vi "Measurement Template.vi"(8 "error in (no error)":errorcluster, 10 "stop":bool, 11 "measurement configuration":cluster{}) -> (0 "error out":errorcluster, 3 "measurement results":cluster{})   [LabVIEW 2021]
uses:
  <vilib>/gRPC/LabVIEW gRPC Library/grpc-lvsupport-release.lvlib
  Runtime/Clients/Measurement Service Client V2/Measurement Service Client V2.lvlib
  35f71eb9-7158-4110-bfb1-6d749e6fa8f4.vi
  Runtime/Clients/Measurement Client V2/Client.lvlib
  ef0035e8-05ef-469b-9be2-5e457b1f40d8.vi
  Runtime/Clients/Measurement Service Client V2/RPC Messages/ni_measurementlink_measurement_v2_MeasureRequest.ctl
  Runtime/Clients/Measurement Service Client V2/RPC Messages/ni_measurementlink_PinMapContext.ctl
  Runtime/Clients/Measurement Service Client V2/RPC Messages/google_protobuf_Any.ctl
panel:
  in  "service class":string="Voltage Measurement_LabVIEW"
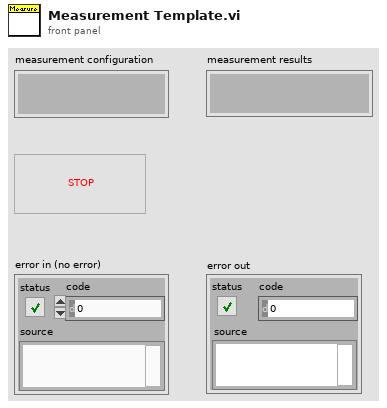
[diagram p1: front panel]
types:
  T1 = typedef "Measurement Service Client V2.lvlib/ni_measurementlink_measurement_v2_MeasureRequest.ctl" = cluster{"configuration_parameters":T2, "pin_map_context":T3}
  T2 = typedef "Measurement Service Client V2.lvlib/google_protobuf_Any.ctl" = cluster{"type_url":string, "value":u8[]}
  T3 = typedef "Measurement Service Client V2.lvlib/ni_measurementlink_PinMapContext.ctl" = cluster{"pin_map_id":string, "sites":i32[]}
  T4 = typedef "grpc-lvsupport-release.lvlib/grpcId.ctl" = u64
  T5 = typedef "grpc-lvsupport-release.lvlib/Message Metadata.ctl" = cluster{"Version":i32, "Name":string, "Type Url":string, "Elements":T6[], "Has Oneof":bool}
  T6 = typedef "grpc-lvsupport-release.lvlib/Message Element Metadata.ctl" = cluster{"Field Name":string, "Embedded Message Name":string, "Protobuf Index":i32, "MessageElementType":T7, "Repeated":bool, "Is in Oneof":bool, "Oneof Container Name":string}
  T7 = typedef "grpc-lvsupport-release.lvlib/Message Element Type.ctl" = enum32{"Int32Value", "FloatValue", "DoubleValue", "BoolValue", "StringValue", "MessageValue", "Int64Value", "UInt32Value", "UInt64Value", "EnumValue", "Bytes", "Fixed64", "Fixed32", "SFixed64", "SFixed32", "SInt64", "SInt32"}
  T8 = typedef "grpc-lvsupport-release.lvlib/Any.ctl" = cluster{"Type Url":string, "Bytes":u8[]}
  T9 = typedef "Measurement Service Client V2.lvlib/ni_measurementlink_measurement_v2_MeasureResponse.ctl" = cluster{"outputs":T2}
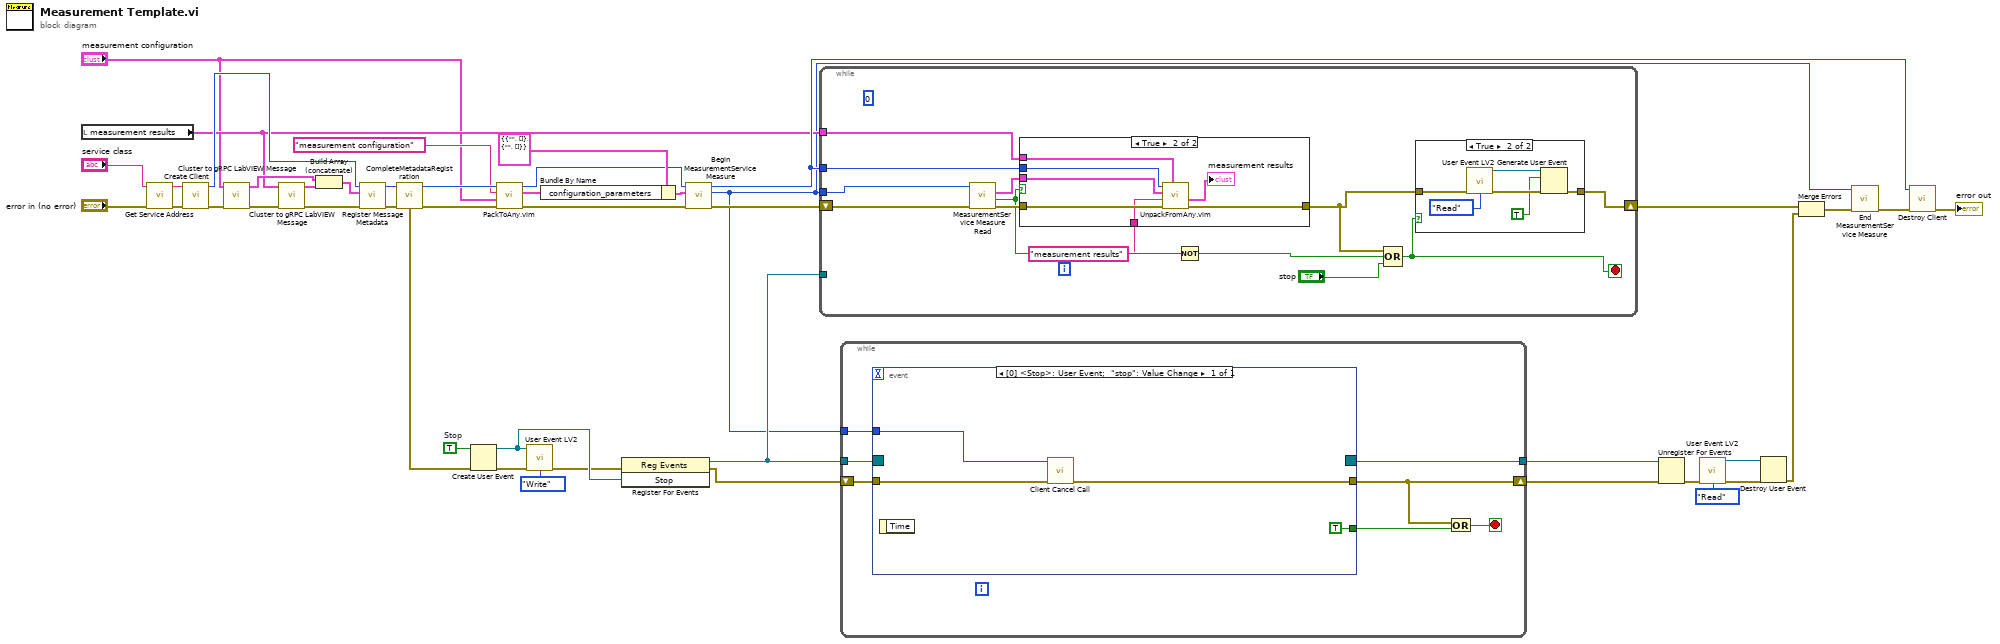
[diagram p0: block diagram]
diagram:
  w20 = TRUE  # Stop
  n1 = local read "measurement results"() -> (w22:cluster{})
  n2 = call "Get Service Address.vi"("error in"="error in (no error)", "service to run"="service class") -> ("error out"=w34:errorcluster, "service address"=w32:string)  [unwired: 8 in]
  n3 = call "Create Client.vi"("error in"=w34, "address"=w32) -> ("error out"=w31:errorcluster, "gRPC ID Out"=w30:T4)  [unwired: 8 in]
  n4 = call <vilib>:"Cluster to gRPC LabVIEW Message.vi"("error in"=w31, "Cluster"="measurement configuration") -> ("error out"=w36:errorcluster, "gRPC Message Metadata []"=w44:T5[])  [unwired: 7 in, 1 out]
  n5 = call <vilib>:"Cluster to gRPC LabVIEW Message.vi"("error in"=w36, "Cluster"=w22) -> ("error out"=w35:errorcluster, "gRPC Message Metadata []"=w43:T5[])  [unwired: 7 in, 1 out]
  n6 = Build Array (concatenate)(w44, w43) -> (w42:T5[])
  n7 = call <vilib>:"Register Message Metadata.vi"("error in"=w35, "Messages"=w42, "gRPCid in"=w30) -> ("error out"=w41:errorcluster, "gRPCid out"=w29:T4)  [unwired: 7 in]
  n8 = call <vilib>:"CompleteMetadataRegistration.vi"("error in"=w41, "gRPC ID in"=w29) -> ("error out"=w19:errorcluster, "gRPC ID Out"=w28:T4)  [unwired: 8 in]
  n9 = Create User Event(user event datatype=w20, error in=w19) -> (user event=w16:refnum<user-event>, error out=w14:errorcluster)
  n10 = call "PackToAny.vim"("error in"=w19, "Data To Pack"="measurement configuration", "Message Type"="measurement configuration", "gRPCid in"=w28) -> ("error out"=w40:errorcluster, "Any"=w38:T8, "gRPCid out"=w24:u64)  [unwired: 5 in]
  n11 = call "User Event LV2.vi"("Stop event"=w16, "error in (no error)"=w14, "LV2 operations"=enum16{"Read", "Write"}."Write") -> ("error out"=w15:errorcluster)  [unwired: 11 in, 1 out]
  n12 = Bundle By Name(cluster=T1 {"configuration_parameters"={"type_url"="", "value"=[]}, "pin_map_context"={"pin_map_id"="", "sites"=[]}} ("Request Data"), "configuration_parameters"=w38) -> (w37:T1)
  n13 = register-events(error in=w15, w16) -> (reference out=w9:refnum<event-registration>, error out=w8:errorcluster)  [unwired: 1 in]
  n14 = call "Begin MeasurementService Measure.vi"("error in"=w40, "Request Data"=w37, "gRPC ID"=w24) -> ("error out"=w18:errorcluster, "Call Id Out"=w2:T4, "gRPC ID out"=w25:T4)  [unwired: 6 in]
  n15 = while {
    tunnel: w2 -> [w56]
    tunnel: w25 -> [w55]
    shift-right: [w45] -> w5
    shift-left: w18 -> [w57]
    tunnel: w22 -> [w54]
    tunnel: w9 -> [_]
    stop <- w47 stop-if-true
    (unwired) 0
    n16 = call "MeasurementService Measure Read.vi"("error in"=w57, "Call ID in"=w56) -> ("error out"=w50:errorcluster, "Success"=w49:bool, "Response Data"=w51:T9)  [unwired: 6 in, 1 out]
    n17 = case shown="True" w49 {
      tunnel: w51 -> [_ w72]
      tunnel: w55 -> [_ w71]
      tunnel: w50 -> [w65 w70]
      tunnel: [w65 w69] -> w46
      tunnel: w54 -> [_ w68]
      tunnel: "measurement results" ("Message Type") -> [_ w67]
      frame False {
      }
      frame True {
        n18 = call "UnpackFromAny.vim"("Data Type"=w68, "error in"=w70, "Message Type"=w67, "Any"=w72, "gRPCid in"=w71) -> ("error out"=w69:errorcluster, "Unpacked Value"=→"measurement results":cluster{"Measurement from SMU Str 2":string})  [unwired: 4 in, 1 out]
      }
    }
    n19 = Not(x=w49) -> (.not. x?=w52:bool)
    n20 = Compound Arithmetic op=OR(w46, w52, "stop") -> (w47:bool)
    n21 = case shown="True" w47 {
      tunnel: w46 -> [w58 w60]
      tunnel: [w58 w59] -> w45
      frame False {
      }
      frame True {
        n22 = call "User Event LV2.vi"("error in (no error)"=w60, "LV2 operations"=enum16{"Read", "Write"}."Read") -> ("Stop event out"=w63:refnum<user-event>, "error out"=w64:errorcluster)  [unwired: 12 in]
        n23 = Generate User Event(user event=w63, event data cluster=TRUE ("event data"), error in=w64) -> (error out=w59:errorcluster)  [unwired: 1 in, 1 out]
      }
    }
  }
  n24 = while {
    shift-right: [w78] -> w7
    shift-left: w8 -> [w79]
    tunnel: [w76] -> w6
    tunnel: w9 -> [w74]
    tunnel: w2 -> [w73]
    stop <- w75 stop-if-true
    n25 = event shown="[0] <Stop>: User Event;  \"stop\": Value Change" {
      selector: w74 -> [_]
      dyn-events: [_] -> w76
      timeout: _ -> [_]
      tunnel: w79 -> [w83]
      tunnel: [w82] -> w78
      tunnel: [TRUE] -> w77
      tunnel: w73 -> [w80]
      event User Event; "stop": Value Change {
        n26 = event-data() -> ()  [unwired: 1 in, 1 out]
        n27 = call <vilib>:"Client Cancel Call.vi"("error in"=w83, "Call ID in"=w80) -> ("error out"=w82:errorcluster)  [unwired: 7 in, 2 out]
      }
    }
    n28 = Compound Arithmetic op=OR(w78, w77) -> (w75:bool)
  }
  n29 = Unregister For Events(event registration refnum=w6, error in=w7) -> (error out=w10:errorcluster)
  n30 = call "User Event LV2.vi"("error in (no error)"=w10, "LV2 operations"=enum16{"Read", "Write"}."Read") -> ("Stop event out"=w12:refnum<user-event>, "error out"=w11:errorcluster)  [unwired: 12 in]
  n31 = Destroy User Event(user event=w12, error in=w11) -> (error out=w3:errorcluster)
  n32 = Merge Errors(w5, w3) -> (w4:errorcluster)
  n33 = call "End MeasurementService Measure.vi"("error in"=w4, "Call ID in"=w2) -> ("error out"=w26:errorcluster)  [unwired: 8 in, 1 out]
  n34 = call "Destroy Client.vi"("error in"=w26, "gRPC ID"=w25) -> ("error out"=→"error out":errorcluster)  [unwired: 9 in]
